vi "Configure Panel.vi"(7 "Console Log in":refnum<class "Console Log.lvclass">, 8 "error in":errorcluster, 11 "Gluing Procedure in":refnum<class "Gluing Procedure.lvclass">) -> (0 "error out":errorcluster, 1 "Cancel Button status":bool, 3 "Gluing Procedure out":refnum<class "Gluing Procedure.lvclass">, 5 "Console Log out":refnum<class "Console Log.lvclass">)   [LabVIEW 2017]
uses:
  Procedure Classes/Gluing Procedure/Gluing Procedure.lvclass
  Shared Components/WorkTable Class/WorkTable Class.lvclass
  UI typedefs/HDI Slot Control.ctl
  UI typedefs/HDI Chuck Control.ctl
  Shared Components/Config Manager Class/Type Definitions/Stamp Type.ctl
  UI typedefs/Stamp Slot Control.ctl
  UI typedefs/Stamp Chuck Control.ctl
  UI typedefs/Glue Slot Control.ctl
  UI typedefs/Glue Chuck Control.ctl
  Shared Components/Config Manager Class/Type Definitions/Weight Type.ctl
  UI typedefs/Weight Slot Control.ctl
  UI typedefs/Weight Chuck Control.ctl
  UI typedefs/BM Slot Control.ctl
  UI typedefs/BM Chuck Control.ctl
  UI typedefs/Active Paths.ctl
  UI typedefs/Glue Path.ctl
  UI typedefs/Glue Paths.ctl
  Procedure Classes/Gluing Procedure/Type Definitions/Configure.ctl
  UI typedefs/BBM Chuck Used.ctl
  Application Utilities/Console Log/Console Log.lvclass
  UI typedefs/Glue Paths Disable.ctl
panel:
  out "Active Paths":T1=[TRUE, TRUE, TRUE, TRUE]
  in  "Set all OFF":bool
  in  "Set all ON":bool
  in  "Glue Pathways":T2=[{"HDI Slot "=0, "Stamp Slot"=0, "Glue Slot"=0, "Weight Slot"=0, "BBM Slot"=0}, {"HDI Slot "=1, "Stamp Slot"=1, "Glue Slot"=1, "Weight Slot"=1, "BBM Slot"=1}, {"HDI Slot "=2, "Stamp Slot"=2, "Glue Slot"=2, "Weight Slot"=2, "BBM Slot"=2}, {"HDI Slot "=3, "Stamp Slot"=3, "Glue Slot"=3, "Weight Slot"=3, "BBM Slot"=3}] {"BBM Slot" items=["Slot 1", "Slot 2", "Slot 3", "Slot 4"]; "Weight Slot" items=["Slot 1", "Slot 2", "Slot 3", "Slot 4"]; "Glue Slot" items=["Slot 1", "Slot 2", "Slot 3", "Slot 4"]; "Stamp Slot" items=["Slot 1", "Slot 2", "Slot 3", "Slot 4"]; "HDI Slot" items=["Slot 1", "Slot 2", "Slot 3", "Slot 4"]}
  in  "HDI Chuck Control":T4
  in  "BBM Chuck Control":T6
  in  "Weight Chuck Control":T8={"Slot 1"={"Populated?"=FALSE, "Weight Type"=enum."Weight 1"}, "Slot 2"={"Populated?"=FALSE, "Weight Type"=enum."Weight 2"}, "Slot 3"={"Populated?"=FALSE, "Weight Type"=enum."Weight 3"}, "Slot 4"={"Populated?"=FALSE, "Weight Type"=enum."Weight 4"}}
  in  "Chuck Module Used for BBM:":T11 items=["Chuck 1", "Chuck 2", "Chuck 3", "Chuck 4"]
  in  "Stamp Chuck Control":T12={"Slot 1"={"Populated?"=FALSE, "Stamp Type"=enum."Stamp 1"}, "Slot 2"={"Populated?"=FALSE, "Stamp Type"=enum."Stamp 2"}, "Slot 3"={"Populated?"=FALSE, "Stamp Type"=enum."Stamp 3"}, "Slot 4"={"Populated?"=FALSE, "Stamp Type"=enum."Stamp 4"}}
  in  "Glue Chuck Control":T15
  in  "Cancel Button":bool
  in  "OK Button":bool
  in  "Path Enabling":T17={"Path 1 BG Color"=65280, "Path 2 BG Color"=65280, "Path 3 BG Color"=65280, "Path 4 BG Color"=65280, "Disable Path 1"=FALSE, "Disable Path 2"=FALSE, "Disable Path 3"=FALSE, "Disable Path 4"=FALSE}
  # "Choose your pathways:"
  # "Procedure:\n1.  Select Chucks that are populated\n2.  Use drop down or text box for identification of element.\n3.  Choose path, as needed."
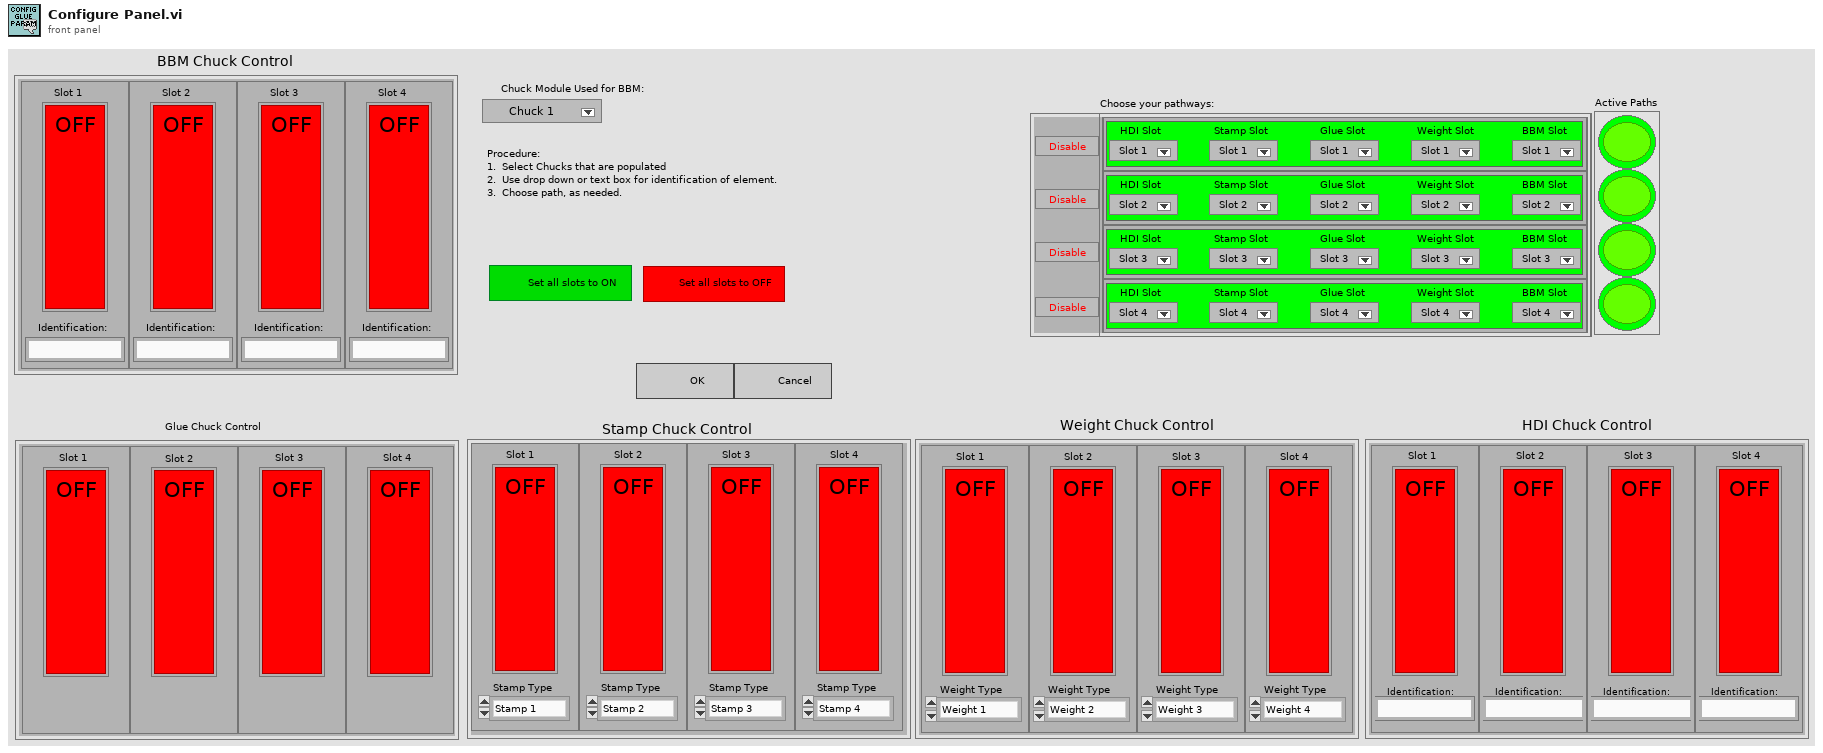
[diagram p1: front panel]
types:
  T1 = typedef "Active Paths.ctl" = bool[]
  T2 = typedef "Glue Paths.ctl" = T3[]
  T3 = typedef "Glue Path.ctl" = cluster{"HDI Slot ":i32, "Stamp Slot":i32, "Glue Slot":i32, "Weight Slot":i32, "BBM Slot":i32}
  T4 = typedef "HDI Chuck Control.ctl" = cluster{"Slot 1":T5, "Slot 2":T5, "Slot 3":T5, "Slot 4":T5}
  T5 = typedef "HDI Slot Control.ctl" = cluster{"Populated?":bool, "Identification:":string}
  T6 = typedef "BM Chuck Control.ctl" = cluster{"Slot 1":T7, "Slot 2":T7, "Slot 3":T7, "Slot 4":T7}
  T7 = typedef "BM Slot Control.ctl" = cluster{"Populated?":bool, "Identification:":string}
  T8 = typedef "Weight Chuck Control.ctl" = cluster{"Slot 1":T9, "Slot 2":T9, "Slot 3":T9, "Slot 4":T9}
  T9 = typedef "Weight Slot Control.ctl" = cluster{"Populated?":bool, "Weight Type":T10}
  T10 = typedef "Weight Type.ctl" = enum16{"Weight 1", "Weight 2", "Weight 3", "Weight 4", "Weight 5", "Weight 6", "Weight 7", "Weight 8", "Weight 9", "Weight 10", "Weight 11", "Weight 12", "Weight 13", "Weight 14", "Weight 15", "Weight 16"}
  T11 = typedef "BBM Chuck Used.ctl" = i32
  T12 = typedef "Stamp Chuck Control.ctl" = cluster{"Slot 1":T13, "Slot 2":T13, "Slot 3":T13, "Slot 4":T13}
  T13 = typedef "Stamp Slot Control.ctl" = cluster{"Populated?":bool, "Stamp Type":T14}
  T14 = typedef "Stamp Type.ctl" = enum16{"Stamp 1", "Stamp 2", "Stamp 3", "Stamp 4", "Stamp 5", "Stamp 6", "Stamp 7", "Stamp 8"}
  T15 = typedef "Glue Chuck Control.ctl" = cluster{"Slot 1":T16, "Slot 2":T16, "Slot 3":T16, "Slot 4":T16}
  T16 = typedef "Glue Slot Control.ctl" = cluster{"Populated?":bool}
  T17 = typedef "Glue Paths Disable.ctl" = cluster{"Path 1 BG Color":u32, "Path 2 BG Color":u32, "Path 3 BG Color":u32, "Path 4 BG Color":u32, "Disable Path 1":bool, "Disable Path 2":bool, "Disable Path 3":bool, "Disable Path 4":bool}
  T18 = enum16{"Empty", "Bare HDI", "Unglued", "Stamped", "PartOnTop", "Weighted", "Unpotted", "Potted"}
  T19 = typedef "Worktable_Weight.ctl" = cluster{"Weight State":enum16{"Empty", "Populated"}, "Weight Type":T10, "Location/Orientation":T20}
  T20 = typedef "Position_Orientation.ctl" = cluster{"Center":refnum<class "Vec3d Class.lvclass">, "Orientation":refnum<class "Orient3d Class.lvclass">}
  T21 = cluster{"Reservoir State":enum16{"Empty", "Full", "Used"}, "Center":refnum<class "Vec3d Class.lvclass">}
  T22 = typedef "Worktable_Stamp.ctl" = cluster{"Stamp State":enum16{"Empty", "Populated", "Used"}, "Location/Orientation":T20, "Stamp Type":T14}
  T23 = typedef "Worktable_Module Slot.ctl" = cluster{"Slot State":enum16{"Empty", "Bare HDI", "Unglued", "Stamped", "PartOnTop", "Weighted", "Unpotted", "Potted"}, "BBM Type":enum16{"None", "BBM", "GlassSlide"}, "HDI Type":enum16{"None", "HDI", "Polyimide"}, "Vacuum Channel":u8, "Location/Orientation BBM":T20, "Location/Orientation HDI":T20, "S/N":string}
  T24 = cluster{"HDI Chuck Control":refnum<vi>, "Stamp Chuck Control":refnum<vi>, "Glue Chuck Control":refnum<vi>, "Weight Chuck Control":refnum<vi>, "BBM Chuck Control":refnum<vi>}
  T25 = typedef "Configure.ctl" = cluster{"Has been run?":bool, "Active Paths":T1, "Glue Pathways":T2, "Chuck Module Used for BBM:":T11}
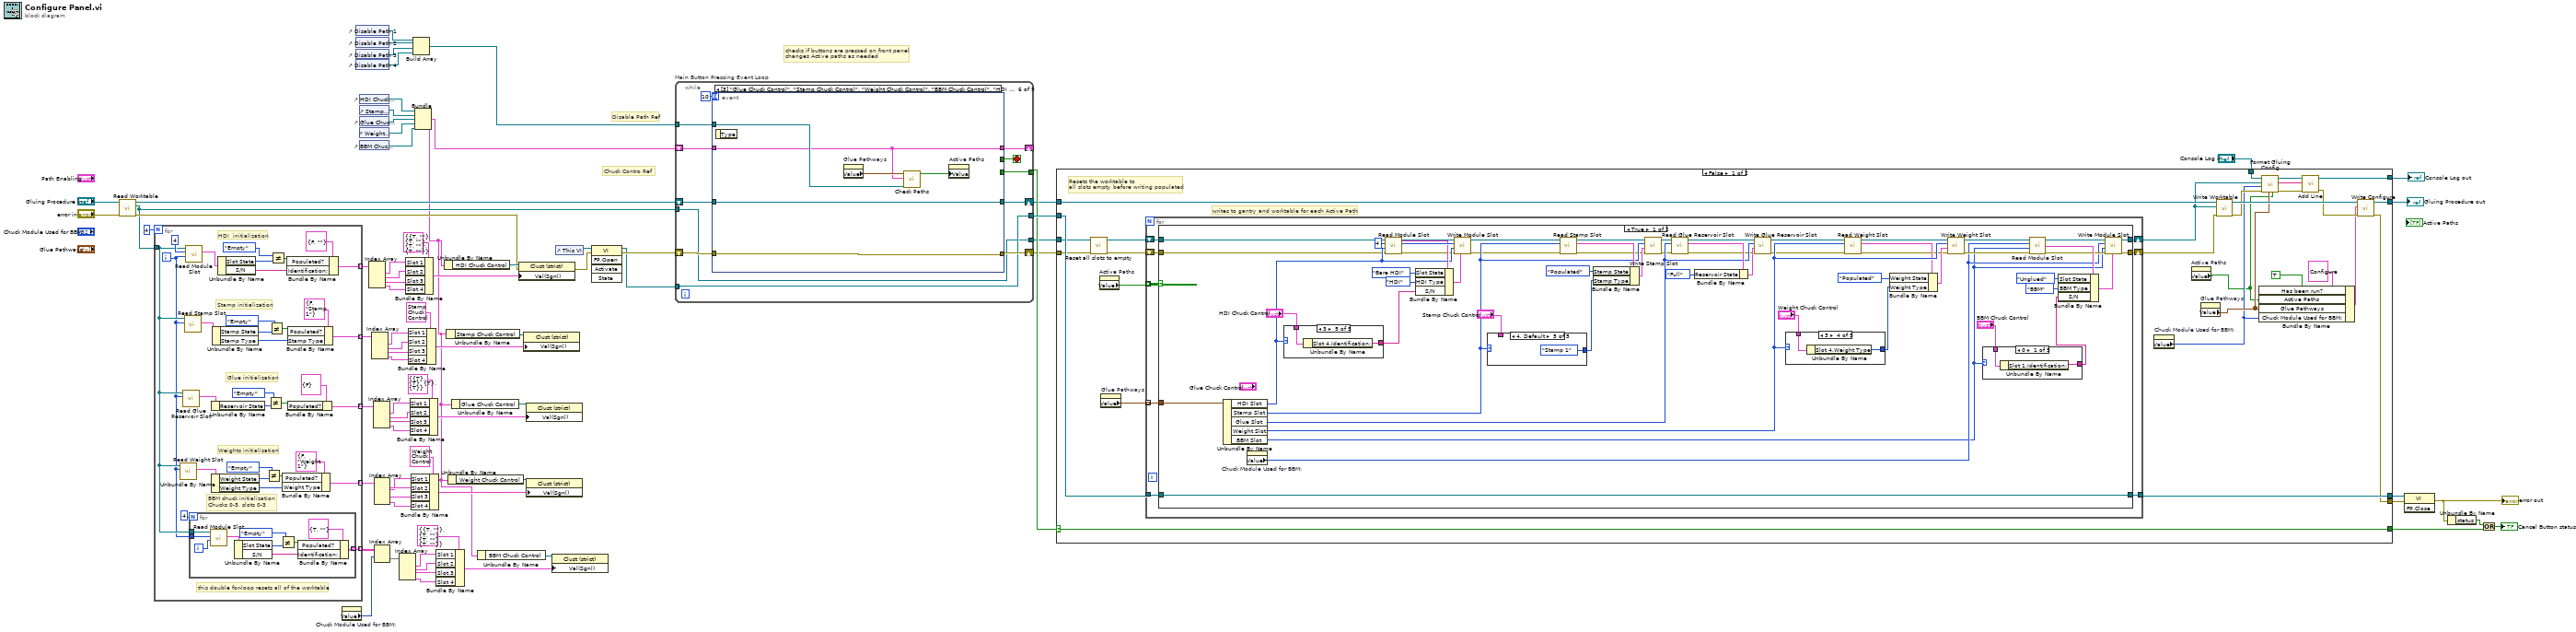
[diagram p0: block diagram]
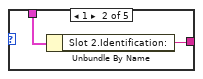
[diagram p2: hidden frame]
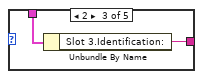
[diagram p3: hidden frame]
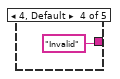
[diagram p4: hidden frame]
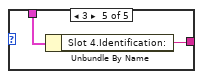
[diagram p5: hidden frame]
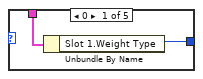
[diagram p6: hidden frame]
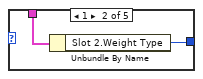
[diagram p7: hidden frame]
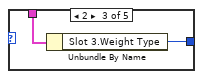
[diagram p8: hidden frame]
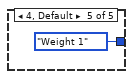
[diagram p9: hidden frame]
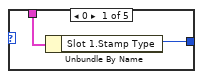
[diagram p10: hidden frame]
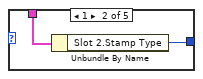
[diagram p11: hidden frame]
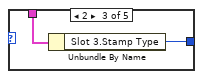
[diagram p12: hidden frame]
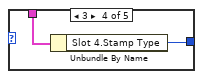
[diagram p13: hidden frame]
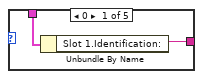
[diagram p14: hidden frame]
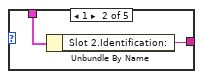
[diagram p15: hidden frame]
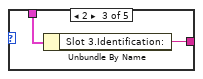
[diagram p16: hidden frame]
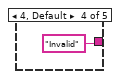
[diagram p17: hidden frame]
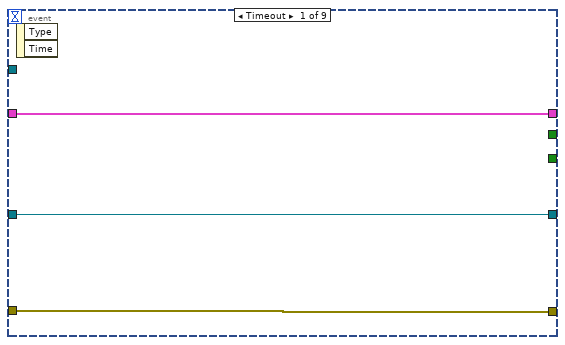
[diagram p20: hidden frame]
diagram:
  # "Chuck Contro Ref"
  # "Disable Path Ref"
  # "checks if buttons are pressed on front panel\nchanges Active paths as needed"
  n1 = call "Read Worktable.vi"("error in"="error in", "Gluing Procedure in"="Gluing Procedure in") -> ("error out"=w10:errorcluster, "WorkTable out"=w7:refnum<class "WorkTable Class.lvclass">, "Gluing Procedure out"=w33:refnum<class "Gluing Procedure.lvclass">)  [unwired: 7 in]
  n2 = for {
    N: 4 -> [_]
    tunnel: [w102] -> w70 mode=indexing
    tunnel: w7 -> [w82]
    tunnel: [w96] -> w13 mode=indexing
    tunnel: [w90] -> w12 mode=indexing
    tunnel: [w84] -> w11 mode=indexing
    tunnel: [w81] -> w4 mode=indexing
    i -> [w80]
    # "this double for-loop resets all of the worktable"
    # "BBM chuck initialization\nChucks 0-3, slots 0-3"
    # "Weights initialization"
    # "Glue initialization"
    # "HDI  initialization"
    # "Stamp initialization"
    n3 = call "Read Weight Slot.vi"("weight slot"=w80, "WorkTable Class in"=w82) -> ("Weight Slot"=w85:T19)  [unwired: 7 in, 2 out]
    n4 = call "Read Glue Reservoir Slot.vi"("index"=w80, "WorkTable Class in"=w82) -> ("Glue Resivoir Slot"=w91:T21)  [unwired: 7 in, 2 out]
    n5 = call "Read Stamp Slot.vi"("Stamp Slot"=w80, "WorkTable Class in"=w82) -> ("Stamp Slot"=w97:T22)  [unwired: 7 in, 2 out]
    n6 = call-dynamic "Read Module Slot.vi"("slot"=w80, "chuck"=4, "WorkTable in"=w82) -> ("Module Slot"=w109:T23)  [unwired: 6 in, 2 out]
    n7 = for {
      N: 4 -> [_]
      tunnel: w82 -> [w116]
      tunnel: [w115] -> w81 mode=indexing
      tunnel: w80 -> [w111]
      i -> [w112]
      n8 = call-dynamic "Read Module Slot.vi"("slot"=w112, "chuck"=w111, "WorkTable in"=w116) -> ("Module Slot"=w119:T23)  [unwired: 6 in, 2 out]
      n9 = Unbundle By Name(w119) -> ("Slot State"=w118:T18, "S/N"=w110:string)
      n10 = Not Equal?(x=T18."Empty", y=w118) -> (x != y?=w117:bool)
      n11 = Bundle By Name(cluster=T7 {"Populated?"=TRUE, "Identification:"=""} ("BBM Slot"), "Populated?"=w117, "Identification:"=w110) -> (w115:T7)
    }
    n12 = Unbundle By Name(w85) -> ("Weight State"=w86:enum16{"Empty", "Populated"}, "Weight Type"=w79:T10)
    n13 = Unbundle By Name(w91) -> ("Reservoir State"=w92:enum16{"Empty", "Full", "Used"})
    n14 = Unbundle By Name(w97) -> ("Stamp State"=w98:enum16{"Empty", "Populated", "Used"}, "Stamp Type"=w78:T14)
    n15 = Unbundle By Name(w109) -> ("Slot State"=w108:T18, "S/N"=w103:string)
    n16 = Not Equal?(x=enum16{"Empty", "Populated"}."Empty", y=w86) -> (x != y?=w87:bool)
    n17 = Not Equal?(x=enum16{"Empty", "Full", "Used"}."Empty", y=w92) -> (x != y?=w93:bool)
    n18 = Not Equal?(x=enum16{"Empty", "Populated", "Used"}."Empty", y=w98) -> (x != y?=w99:bool)
    n19 = Not Equal?(x=T18."Empty", y=w108) -> (x != y?=w105:bool)
    n20 = Bundle By Name(cluster=T9 {"Populated?"=FALSE, "Weight Type"=enum."Weight 1"} ("Weight Slot"), "Populated?"=w87, "Weight Type"=w79) -> (w84:T9)
    n21 = Bundle By Name(cluster=T5 {"Populated?"=FALSE, "Identification:"=""} ("Chuck"), "Populated?"=w105, "Identification:"=w103) -> (w102:T5)
    n22 = Bundle By Name(cluster=T13 {"Populated?"=FALSE, "Stamp Type"=enum."Stamp 1"} ("Stamp Slot"), "Populated?"=w99, "Stamp Type"=w78) -> (w96:T13)
    n23 = Bundle By Name(cluster=T16 {"Populated?"=FALSE} ("Glue Slot"), "Populated?"=w93) -> (w90:T16)
  }
  n24 = property on="Chuck Module Used for BBM:" class="Ring (strict)"() -> ("Value"=w2:T11)  [unwired: 2 in, 2 out]
  n25 = control-ref of="Disable Path 1"() -> (w18:refnum<vi>)
  n26 = control-ref of="Disable Path 2"() -> (w17:refnum<vi>)
  n27 = control-ref of="Disable Path 3"() -> (w16:refnum<vi>)
  n28 = control-ref of="Disable Path 4"() -> (w15:refnum<vi>)
  n29 = control-ref of="BBM Chuck Control"() -> (w5:refnum<vi>)
  n30 = control-ref of="HDI Chuck Control"() -> (w76:refnum<vi>)
  n31 = control-ref of="Stamp Chuck Control"() -> (w75:refnum<vi>)
  n32 = control-ref of="Glue Chuck Control"() -> (w74:refnum<vi>)
  n33 = control-ref of="Weight Chuck Control"() -> (w73:refnum<vi>)
  n34 = Index Array(array=w70) -> (element #1=w68:T5, element #2=w67:T5, element #3=w66:T5, element #4=w65:T5)  [unwired: 4 in]
  n35 = Index Array(array=w13) -> (element #1=w59:T13, element #2=w60:T13, element #3=w61:T13, element #4=w62:T13)  [unwired: 4 in]
  n36 = Index Array(array=w12) -> (element #1=w53:T16, element #2=w52:T16, element #3=w51:T16, element #4=w50:T16)  [unwired: 4 in]
  n37 = Index Array(array=w11) -> (element #1=w42:T9, element #2=w43:T9, element #3=w44:T9, element #4=w45:T9)  [unwired: 4 in]
  n38 = Index Array(array=w4, index (row)=w2) -> (element=w3:T7[])  [unwired: 1 in]
  n39 = Index Array(array=w3) -> (element #1=w40:T7, element #2=w39:T7, element #3=w38:T7, element #4=w37:T7)  [unwired: 4 in]
  n40 = Bundle By Name(cluster=T4 {"Slot 1"={"Populated?"=TRUE, "Identification:"=""}, "Slot 2"={"Populated?"=TRUE, "Identification:"=""}, "Slot 3"={"Populated?"=TRUE, "Identification:"=""}, "Slot 4"={"Populated?"=TRUE, "Identification:"=""}} ("HDI Chuck Control"), "Slot 1"=w68, "Slot 2"=w67, "Slot 3"=w66, "Slot 4"=w65) -> (w63:T4)
  n41 = Bundle By Name(cluster=T12 {"Slot 1"={"Populated?"=TRUE, "Stamp Type"=enum."Stamp 1"}, "Slot 2"={"Populated?"=TRUE, "Stamp Type"=enum."Stamp 2"}, "Slot 3"={"Populated?"=TRUE, "Stamp Type"=enum."Stamp 3"}, "Slot 4"={"Populated?"=TRUE, "Stamp Type"=enum."Stamp 4"}} ("Stamp Chuck Control"), "Slot 1"=w59, "Slot 2"=w60, "Slot 3"=w61, "Slot 4"=w62) -> (w56:T12)
  n42 = Bundle By Name(cluster=T15 {"Slot 1"={"Populated?"=TRUE}, "Slot 2"={"Populated?"=TRUE}, "Slot 3"={"Populated?"=TRUE}, "Slot 4"={"Populated?"=TRUE}} ("Glue Chuck Control"), "Slot 1"=w53, "Slot 2"=w52, "Slot 3"=w51, "Slot 4"=w50) -> (w48:T15)
  n43 = Bundle By Name(cluster=T8 {"Slot 1"={"Populated?"=TRUE, "Weight Type"=enum."Weight 1"}, "Slot 2"={"Populated?"=TRUE, "Weight Type"=enum."Weight 2"}, "Slot 3"={"Populated?"=TRUE, "Weight Type"=enum."Weight 3"}, "Slot 4"={"Populated?"=TRUE, "Weight Type"=enum."Weight 4"}} ("Weight Chuck Control"), "Slot 1"=w42, "Slot 2"=w43, "Slot 3"=w44, "Slot 4"=w45) -> (w47:T8)
  n44 = Build Array(w18, w17, w16, w15) -> (w14:refnum<vi>[])
  n45 = Bundle("HDI Chuck Control"=w76, "Stamp Chuck Control"=w75, "Glue Chuck Control"=w74, "Weight Chuck Control"=w73, "BBM Chuck Control"=w5) -> (w1:T24)  [unwired: 1 in]
  n46 = Bundle By Name(cluster=T6 {"Slot 1"={"Populated?"=TRUE, "Identification:"=""}, "Slot 2"={"Populated?"=TRUE, "Identification:"=""}, "Slot 3"={"Populated?"=TRUE, "Identification:"=""}, "Slot 4"={"Populated?"=TRUE, "Identification:"=""}} ("BM Chuck Control"), "Slot 1"=w40, "Slot 2"=w39, "Slot 3"=w38, "Slot 4"=w37) -> (w35:T6)
  n47 = Unbundle By Name(w1) -> ("HDI Chuck Control"=w64:refnum<vi>)
  n48 = Unbundle By Name(w1) -> ("Stamp Chuck Control"=w57:refnum<vi>)
  n49 = Unbundle By Name(w1) -> ("Weight Chuck Control"=w46:refnum<vi>)
  n50 = Unbundle By Name(w1) -> ("Glue Chuck Control"=w49:refnum<vi>)
  n51 = Unbundle By Name(w1) -> ("BBM Chuck Control"=w36:refnum<vi>)
  n52 = property class="Clust (strict)"(reference=w64, error in=w10, "Val(Sgnl)"=w63) -> (error out=w9:errorcluster)  [unwired: 1 out]
  n53 = property class="Clust (strict)"(reference=w57, "Val(Sgnl)"=w56) -> ()  [unwired: 1 in, 2 out]
  n54 = property class="Clust (strict)"(reference=w49, "Val(Sgnl)"=w48) -> ()  [unwired: 1 in, 2 out]
  n55 = property class="Clust (strict)"(reference=w46, "Val(Sgnl)"=w47) -> ()  [unwired: 1 in, 2 out]
  n56 = property class="Clust (strict)"(reference=w36, "Val(Sgnl)"=w35) -> ()  [unwired: 1 in, 2 out]
  n57 = control-ref of="This VI"() -> (w77:refnum<vi>)
  n58 = invoke class="VI" method="FP.Open"(reference=w77, error in=w9) -> (reference out=w8:refnum<vi>, error out=w32:errorcluster)  [unwired: 3 in, 3 out]
  n59 = while "Main Button Pressing Event Loop" {
    tunnel: [w123] -> w31
    shift-right: [w129] -> w26
    shift-left: w32 -> [w130]
    shift-right: [w127] -> w28
    shift-left: w33 -> [w128]
    tunnel: [w125] -> w29
    tunnel: w14 -> [w124]
    tunnel: w8 -> [w123]
    tunnel: w7 -> [w122]
    tunnel: [w122] -> w6
    shift-right: [w120] -> _
    shift-left: w1 -> [w121]
    stop <- w126 stop-if-true
    n60 = event shown="[5] \"Glue Chuck Control\", \"Stamp Chuck Control\", \"Weight Chuck Control\", \"BBM Chuck Control\", \"HDI Chuck Control\": Value Change" {
      selector: _ -> [_ _ _ _ _ _ _ _ _]
      dyn-events: _ -> [_ _ _ _ _ _ _ _ _]
      timeout: 10 -> [_ _ _ _ _ _ _ _ _]
      tunnel: [_ w139 w146 _ _ _ _ _ _] -> w126
      tunnel: w121 -> [w132 w135 w145 w152 w160 w161 w167 w173 w213]
      tunnel: w130 -> [w134 w140 w147 w150 w156 w165 w171 w175 w214]
      tunnel: [w134 w140 w147 w149 w155 w165 w171 w175 w214] -> w129
      tunnel: w128 -> [w133 w141 w148 w153 w158 w166 w172 w174 w215]
      tunnel: [w133 w141 w148 w153 w158 w166 w172 w174 w215] -> w127
      tunnel: [_ _ w146 _ _ _ _ _ _] -> w125
      tunnel: w124 -> [_ _ _ _ _ w163 w169 w176 _]
      tunnel: [w132 w135 w145 w151 w157 w161 w167 w173 w213] -> w120
      event Timeout {
        n61 = event-data() -> ()  [unwired: 1 in, 2 out]
      }
      event "OK Button": Value Change {
        n62 = event-data() -> ()  [unwired: 1 in, 1 out]
        n63 = property on="Active Paths" class="Arr (strict)"() -> ("Value"=w138:T1)  [unwired: 2 in, 2 out]
        n64 = call "Number of Active Paths.vi"("Active Paths"=w138) -> ("Number of Active Paths"=w137:i32)  [unwired: 10 in]
        n65 = Greater Than 0?(x=w137) -> (x > 0?=w136:bool)
        n66 = case shown="False" w136 {
          tunnel: [FALSE TRUE] -> w139
          frame False {
            n67 = One Button Dialog(message="No active paths are\nenabled.  Please choose\nan active path to continue.") -> ()  [unwired: 1 in, 1 out]
          }
          frame True {
          }
        }
      }
      event "Cancel Button": Value Change {
        w146 = TRUE
        n68 = event-data() -> ()  [unwired: 1 in, 5 out]
      }
      event "Set all ON": Mouse Up {
        n69 = event-data() -> ()  [unwired: 1 in, 1 out]
        n70 = call "Set chucks on or off.vi"("error in"=w150, "Populated on/off"=TRUE, "Chuck Control ref in"=w152) -> ("error out"=w149:errorcluster, "Chuck Control ref out"=w151:T24)  [unwired: 7 in]
      }
      event "Set all OFF": Mouse Up {
        n71 = event-data() -> ()  [unwired: 1 in, 1 out]
        n72 = call "Set chucks on or off.vi"("error in"=w156, "Populated on/off"=FALSE, "Chuck Control ref in"=w160) -> ("error out"=w155:errorcluster, "Chuck Control ref out"=w157:T24)  [unwired: 7 in]
      }
      event Value Change {
        n73 = event-data() -> ()  [unwired: 1 in, 1 out]
        n74 = property on="Glue Pathways" class="Arr (strict)"() -> ("Value"=w164:T2)  [unwired: 2 in, 2 out]
        n75 = call "Check Paths.vi"("Path Disabled Ref"=w163, "Chuck Control ref in"=w161, "Glue Pathways"=w164) -> ("Active Paths"=w162:T1)  [unwired: 8 in]
        n76 = property on="Active Paths" class="Arr (strict)"("Value"=w162) -> ()  [unwired: 2 in, 2 out]
      }
      event Value Change {
        n77 = event-data() -> ()  [unwired: 1 in, 1 out]
        n78 = property on="Glue Pathways" class="Arr (strict)"() -> ("Value"=w170:T2)  [unwired: 2 in, 2 out]
        n79 = call "Check Paths.vi"("Path Disabled Ref"=w169, "Chuck Control ref in"=w167, "Glue Pathways"=w170) -> ("Active Paths"=w168:T1)  [unwired: 8 in]
        n80 = property on="Active Paths" class="Arr (strict)"("Value"=w168) -> ()  [unwired: 2 in, 2 out]
      }
      event Value Change {
        n81 = event-data() -> ("CtlRef"=w177:refnum<vi>, "NewVal"=w178:bool)  [unwired: 1 in, 3 out]
        n82 = case shown="False" w178 {
          tunnel: w177 -> [w181 w198]
          tunnel: w177 -> [w180 w197]
          tunnel: w176 -> [w179 w196]
          frame True {
            n83 = for {
              tunnel: w179 -> [w185] mode=indexing
              tunnel: w180 -> [w186]
              i -> [w183]
              n84 = Equal?(x=w185, y=w186) -> (x = y?=w184:bool)
              n85 = case shown="True" w184 {
                tunnel: w183 -> [_ w187]
                frame False {
                }
                frame True {
                  n86 = call <vilib>:"RGB to Color.vi"("B"=u8 0, "G"=u8 0, "R"=u8 255) -> ("Color"=w191:u32)
                  n87 = case shown="3" w187 {
                    tunnel: w191 -> [w192 w193 w194 w195 _]
                    frame 0 {
                      n88 = property on="Path 1 BG Color" class="ColBox"("Val(Sgnl)"=w192) -> ()  [unwired: 2 in, 2 out]
                    }
                    frame 1 {
                      n89 = property on="Path 2 BG Color" class="ColBox"("Val(Sgnl)"=w193) -> ()  [unwired: 2 in, 2 out]
                    }
                    frame 2 {
                      n90 = property on="Path 3 BG Color" class="ColBox"("Val(Sgnl)"=w194) -> ()  [unwired: 2 in, 2 out]
                    }
                    frame 3 {
                      n91 = property on="Path 4 BG Color" class="ColBox"("Val(Sgnl)"=w195) -> ()  [unwired: 2 in, 2 out]
                    }
                    frame 4, Default {
                    }
                  }
                }
              }
            }
            n92 = property class="Bool (strict)"(reference=w181, "BoolText.Text"="Enable" ("Label.Text")) -> ()  [unwired: 1 in, 2 out]
          }
          frame False {
            n93 = for {
              tunnel: w196 -> [w202] mode=indexing
              tunnel: w197 -> [w203]
              i -> [w200]
              n94 = Equal?(x=w202, y=w203) -> (x = y?=w201:bool)
              n95 = case shown="True" w201 {
                tunnel: w200 -> [_ w204]
                frame False {
                }
                frame True {
                  n96 = call <vilib>:"RGB to Color.vi"("B"=u8 0, "G"=u8 255, "R"=u8 0) -> ("Color"=w208:u32)
                  n97 = case shown="3" w204 {
                    tunnel: w208 -> [w209 w210 w211 w212 _]
                    frame 0 {
                      n98 = property on="Path 1 BG Color" class="ColBox"("Val(Sgnl)"=w209) -> ()  [unwired: 2 in, 2 out]
                    }
                    frame 1 {
                      n99 = property on="Path 2 BG Color" class="ColBox"("Val(Sgnl)"=w210) -> ()  [unwired: 2 in, 2 out]
                    }
                    frame 2 {
                      n100 = property on="Path 3 BG Color" class="ColBox"("Val(Sgnl)"=w211) -> ()  [unwired: 2 in, 2 out]
                    }
                    frame 3 {
                      n101 = property on="Path 4 BG Color" class="ColBox"("Val(Sgnl)"=w212) -> ()  [unwired: 2 in, 2 out]
                    }
                    frame 4, Default {
                    }
                  }
                }
              }
            }
            n102 = property class="Bool (strict)"(reference=w198, "BoolText.Text"="Disable" ("Label.Text")) -> ()  [unwired: 1 in, 2 out]
          }
        }
      }
      event Panel Close? {
        # "disables the windows X button"
        n103 = event-data() -> ()  [unwired: 1 in, 3 out]
        n104 = event-data("Discard?"=FALSE) -> ()  [unwired: 1 in, 1 out]
      }
    }
  }
  n105 = case shown="False" w29 {
    selector: w29 -> [w240 w349]
    tunnel: w31 -> [w241 w352]
    tunnel: [w242 w352] -> w30
    tunnel: w28 -> [w223 w351]
    tunnel: [w243 w351] -> w27
    tunnel: w26 -> [w220 w350]
    tunnel: [w240 w349] -> w21
    tunnel: [w239 w350] -> w24
    tunnel: "Console Log in" -> [w238 w348]
    tunnel: [w232 w348] -> w19
    tunnel: w6 -> [w222 _]
    frame False {
      # "writes to gantry and worktable for each Active Path"
      # "Resets the worktable to\nall slots empty before writing populated"
      n106 = call "Reset all slots to empty.vi"("error in"=w220, "WorkTable Class in"=w222) -> ("error out"=w219:errorcluster, "WorkTable Class out"=w221:refnum<class "WorkTable Class.lvclass">)  [unwired: 8 in]
      n107 = property on="Active Paths" class="Arr (strict)"() -> ("Value"=w226:T1)  [unwired: 2 in, 2 out]
      n108 = property on="Glue Pathways" class="Arr (strict)"() -> ("Value"=w224:T2)  [unwired: 2 in, 2 out]
      n109 = for {
        tunnel: w226 -> [w252] mode=indexing
        shift-right: [w250] -> w218
        shift-left: w221 -> [w251]
        shift-right: [w249] -> w217
        shift-left: w219 -> [w248]
        tunnel: [w247] -> w242
        tunnel: w241 -> [w246]
        tunnel: w224 -> [w245] mode=indexing
        n110 = case shown="True" w252 {
          tunnel: w251 -> [w308 w346]
          tunnel: [w274 w346] -> w250
          tunnel: [w273 w345] -> w249
          tunnel: w248 -> [w262 w345]
          tunnel: [w261 w347] -> w247
          tunnel: w246 -> [w261 w347]
          tunnel: w245 -> [w256 _]
          frame True {
            w307 = 4 ("chuck")
            n111 = Unbundle By Name(w256) -> ("HDI Slot"=w295:i32, "Stamp Slot"=w294:i32, "Glue Slot"=w288:i32, "Weight Slot"=w285:i32, "BBM Slot"=w254:i32)
            n112 = property on="Chuck Module Used for BBM:" class="Ring (strict)"() -> ("Value"=w257:T11)  [unwired: 2 in, 2 out]
            n113 = case shown="3" w295 {
              tunnel: "HDI Chuck Control" -> [w337 w339 w341 _ w344]
              tunnel: [w336 w338 w340 "Invalid" w343] -> w303
              frame 0 {
                n114 = Unbundle By Name(w337) -> ("Slot 1.Identification:"=w336:string)
              }
              frame 1 {
                n115 = Unbundle By Name(w339) -> ("Slot 2.Identification:"=w338:string)
              }
              frame 2 {
                n116 = Unbundle By Name(w341) -> ("Slot 3.Identification:"=w340:string)
              }
              frame 4, Default {
              }
              frame 3 {
                n117 = Unbundle By Name(w344) -> ("Slot 4.Identification:"=w343:string)
              }
            }
            n118 = call-dynamic "Read Module Slot.vi"("error in"=w262, "slot"=w295, "chuck"=w307, "WorkTable in"=w308) -> ("error out"=w263:errorcluster, "Module Slot"=w306:T23, "WorkTable out"=w302:refnum<class "WorkTable Class.lvclass">)  [unwired: 5 in]
            n119 = Bundle By Name(cluster=w306, "Slot State"=T18."Bare HDI", "HDI Type"=enum16{"None", "HDI", "Polyimide"}."HDI", "S/N"=w303) -> (w264:T23)
            n120 = call-dynamic "Write Module Slot.vi"("Module Slot"=w264, "error in"=w263, "slot"=w295, "chuck"=w307, "WorkTable in"=w302) -> ("error out"=w265:errorcluster, "WorkTable out"=w301:refnum<class "WorkTable Class.lvclass">)  [unwired: 5 in]
            n121 = case shown="4, Default" w294 {
              tunnel: "Stamp Chuck Control" -> [w328 w330 w332 w334 _]
              tunnel: [w327 w329 w331 w333 Stamp_Type."Stamp 1" ("Stamp Type")] -> w296
              frame 0 {
                n122 = Unbundle By Name(w328) -> ("Slot 1.Stamp Type"=w327:T14)
              }
              frame 1 {
                n123 = Unbundle By Name(w330) -> ("Slot 2.Stamp Type"=w329:T14)
              }
              frame 2 {
                n124 = Unbundle By Name(w332) -> ("Slot 3.Stamp Type"=w331:T14)
              }
              frame 3 {
                n125 = Unbundle By Name(w334) -> ("Slot 4.Stamp Type"=w333:T14)
              }
              frame 4, Default {
              }
            }
            n126 = call "Read Stamp Slot.vi"("error in (no error)"=w265, "Stamp Slot"=w294, "WorkTable Class in"=w301) -> ("error out"=w266:errorcluster, "Stamp Slot"=w300:T22, "WorkTable Class out"=w298:refnum<class "WorkTable Class.lvclass">)  [unwired: 6 in]
            n127 = Bundle By Name(cluster=w300, "Stamp State"=enum16{"Empty", "Populated", "Used"}."Populated", "Stamp Type"=w296) -> (w297:T22)
            n128 = call "Write Stamp Slot.vi"("error in (no error)"=w266, 9:"Stamp Slot"=w297, 10:"Stamp Slot"=w294, "WorkTable Class in"=w298) -> ("error out"=w267:errorcluster, "WorkTable Class out"=w293:refnum<class "WorkTable Class.lvclass">)  [unwired: 6 in]
            n129 = call "Read Glue Reservoir Slot.vi"("error in (no error)"=w267, "index"=w288, "WorkTable Class in"=w293) -> ("error out"=w268:errorcluster, "Glue Resivoir Slot"=w292:T21, "WorkTable Class out"=w290:refnum<class "WorkTable Class.lvclass">)  [unwired: 6 in]
            n130 = Bundle By Name(cluster=w292, "Reservoir State"=enum16{"Empty", "Full", "Used"}."Full") -> (w289:T21)
            n131 = call "Write Glue Reservoir Slot.vi"("error in (no error)"=w268, "Glue Resivoir Slot"=w289, "index"=w288, "WorkTable Class in"=w290) -> ("error out"=w269:errorcluster, "WorkTable Class out"=w287:refnum<class "WorkTable Class.lvclass">)  [unwired: 6 in]
            n132 = case shown="3" w285 {
              tunnel: "Weight Chuck Control" -> [w319 w321 w323 w325 _]
              tunnel: [w318 w320 w322 w324 Weight_Type."Weight 1" ("Weight Type")] -> w282
              frame 0 {
                n133 = Unbundle By Name(w319) -> ("Slot 1.Weight Type"=w318:T10)
              }
              frame 1 {
                n134 = Unbundle By Name(w321) -> ("Slot 2.Weight Type"=w320:T10)
              }
              frame 2 {
                n135 = Unbundle By Name(w323) -> ("Slot 3.Weight Type"=w322:T10)
              }
              frame 3 {
                n136 = Unbundle By Name(w325) -> ("Slot 4.Weight Type"=w324:T10)
              }
              frame 4, Default {
              }
            }
            n137 = call "Read Weight Slot.vi"("error in (no error)"=w269, "weight slot"=w285, "WorkTable Class in"=w287) -> ("error out"=w270:errorcluster, "Weight Slot"=w284:T19, "WorkTable Class out"=w286:refnum<class "WorkTable Class.lvclass">)  [unwired: 6 in]
            n138 = Bundle By Name(cluster=w284, "Weight State"=enum16{"Empty", "Populated"}."Populated", "Weight Type"=w282) -> (w281:T19)
            n139 = call "Write Weight Slot.vi"("error in (no error)"=w270, "Weight Slot"=w281, "weight slot"=w285, "WorkTable Class in"=w286) -> ("error out"=w271:errorcluster, "WorkTable Class out"=w277:refnum<class "WorkTable Class.lvclass">)  [unwired: 6 in]
            n140 = case shown="0" w254 {
              tunnel: "BBM Chuck Control" -> [w310 w312 w314 _ w317]
              tunnel: [w309 w311 w313 "Invalid" w316] -> w253
              frame 0 {
                n141 = Unbundle By Name(w310) -> ("Slot 1.Identification:"=w309:string)
              }
              frame 1 {
                n142 = Unbundle By Name(w312) -> ("Slot 2.Identification:"=w311:string)
              }
              frame 2 {
                n143 = Unbundle By Name(w314) -> ("Slot 3.Identification:"=w313:string)
              }
              frame 4, Default {
              }
              frame 3 {
                n144 = Unbundle By Name(w317) -> ("Slot 4.Identification:"=w316:string)
              }
            }
            n145 = call-dynamic "Read Module Slot.vi"("error in"=w271, "slot"=w254, "chuck"=w257, "WorkTable in"=w277) -> ("error out"=w272:errorcluster, "Module Slot"=w278:T23, "WorkTable out"=w280:refnum<class "WorkTable Class.lvclass">)  [unwired: 5 in]
            n146 = Bundle By Name(cluster=w278, "Slot State"=T18."Unglued", "BBM Type"=enum16{"None", "BBM", "GlassSlide"}."BBM", "S/N"=w253) -> (w275:T23)
            n147 = call-dynamic "Write Module Slot.vi"("Module Slot"=w275, "error in"=w272, "slot"=w254, "chuck"=w257, "WorkTable in"=w280) -> ("error out"=w273:errorcluster, "WorkTable out"=w274:refnum<class "WorkTable Class.lvclass">)  [unwired: 5 in]
          }
          frame False {
          }
        }
      }
      n148 = property on="Chuck Module Used for BBM:" class="Ring (strict)"() -> ("Value"=w228:T11)  [unwired: 2 in, 2 out]
      n149 = property on="Active Paths" class="Arr (strict)"() -> ("Value"=w225:T1)  [unwired: 2 in, 2 out]
      n150 = property on="Glue Pathways" class="Arr (strict)"() -> ("Value"=w229:T2)  [unwired: 2 in, 2 out]
      n151 = call "Write Worktable.vi"("error in"=w217, "WorkTable"=w218, "Gluing Procedure in"=w223) -> ("error out"=w235:errorcluster, "Gluing Procedure out"=w244:refnum<class "Gluing Procedure.lvclass">)  [unwired: 7 in]
      n152 = Bundle By Name(cluster=T25 {"Has been run?"=FALSE, "Active Paths"=[TRUE, TRUE, TRUE, TRUE], "Glue Pathways"=[{"HDI Slot "=0, "Stamp Slot"=0, "Glue Slot"=0, "Weight Slot"=0, "BBM Slot"=0}, {"HDI Slot "=1, "Stamp Slot"=1, "Glue Slot"=1, "Weight Slot"=1, "BBM Slot"=1}, {"HDI Slot "=2, "Stamp Slot"=2, "Glue Slot"=2, "Weight Slot"=2, "BBM Slot"=2}, {"HDI Slot "=3, "Stamp Slot"=3, "Glue Slot"=3, "Weight Slot"=3, "BBM Slot"=3}], "Chuck Module Used for BBM:"=0} ("Configure"), "Has been run?"=TRUE, "Active Paths"=w225, "Glue Pathways"=w229, "Chuck Module Used for BBM:"=w228) -> (w227:T25)
      n153 = call "Format Gluing Config.vi"("Active Paths"=w225, "Glue Pathways"=w229, "error in"=w235, "Chuck Module Used for BBM:"=w228, "Worktable"=w218, "Console Log in"=w238) -> ("error out"=w234:errorcluster, "Formatted Worktable Config"=w236:string, "Console Log out"=w237:refnum<class "Console Log.lvclass">)  [unwired: 3 in]
      n154 = call "Add Line.vi"("error in"=w234, "String"=w236, "Console Log in"=w237) -> ("error out"=w233:errorcluster, "Console Log out"=w232:refnum<class "Console Log.lvclass">)  [unwired: 7 in]
      n155 = call "Write Configure.vi"("error in (no error)"=w233, "Configure"=w227, "Gluing Procedure in"=w244) -> ("error out"=w239:errorcluster, "Gluing Procedure out"=w243:refnum<class "Gluing Procedure.lvclass">)  [unwired: 7 in]
    }
    frame True {
    }
  }
  "Gluing Procedure out" <- w27
  "Console Log out" <- w19
  n156 = invoke class="VI" method="FP.Close"(reference=w30, error in=w24) -> (error out=w23:errorcluster)  [unwired: 1 in, 2 out]
  "error out" <- w23
  n157 = Unbundle By Name(w23) -> ("status"=w22:bool)
  n158 = Or(x=w22, y=w21) -> (x .or. y?=→"Cancel Button status":bool)
